vi "Lithographify.vi"(0 "interpolation distance":dbl, 1 "Path Settings.lvclass":refnum<class "Path Settings.lvclass">, 5 "Data In":cluster{string, cluster{"X":dbl, "Y":dbl}[]}, 7 "Direction":u16, 9 "Speed (um/s)":T1={"Schedule"=enum."Constant", "Settings"=variant(dbl 0.0)}, 11 "Voltage (V)":T1={"Schedule"=enum."Constant", "Settings"=variant(dbl 0.0)}, 13 "Enabled":bool) -> (4 "Lithography Data":T3)   [LabVIEW 2019]
doc: "This VI calculates the lithography data of one pattern and organizes it appropriately."
uses:
  typedefs/Voltage - cluster.ctl
  typedefs/Schedule - enum.ctl
  Classes/Settings/Path Settings/Path Settings.lvclass
  typedefs/Schedule Types/Schedule--Formula.ctl
  Classes/Settings/ObjectSettings/ObjectSettings.lvclass
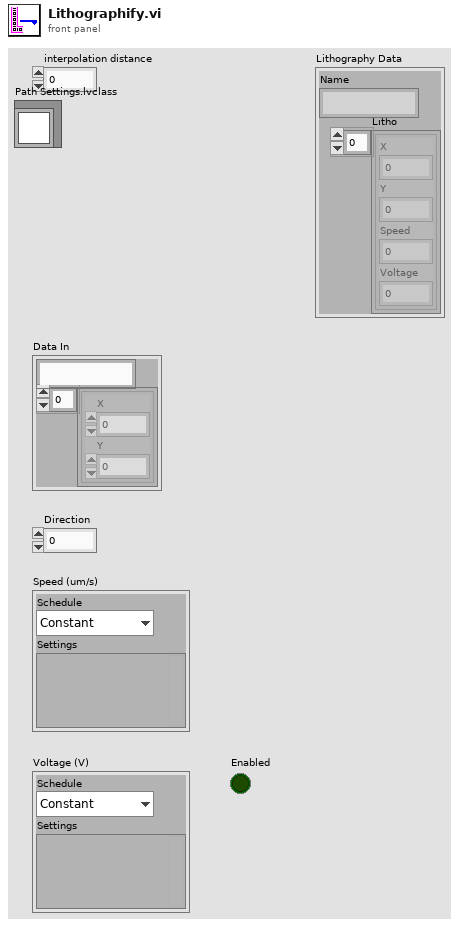
[diagram p1: front panel]
types:
  T1 = typedef "Voltage - cluster.ctl" = cluster{"Schedule":T2, "Settings":variant}
  T2 = typedef "Schedule - enum.ctl" = enum16{"Constant", "Ramp", "Fn. Generator", "Formula"}
  T3 = cluster{"Name":string, "Litho":cluster{"X":dbl, "Y":dbl, "Speed":dbl, "Voltage":dbl}[]}
  T4 = typedef "Schedule--Formula.ctl" = cluster{"formula":string, "formula length (nm)":dbl, "formula resolution (nm)":dbl}
  T5 = cluster{"X":dbl, "Y":dbl, "Speed":dbl, "Voltage":dbl}[]
  T6 = cluster{"X":dbl, "Y":dbl, "Speed":dbl, "Voltage":dbl}
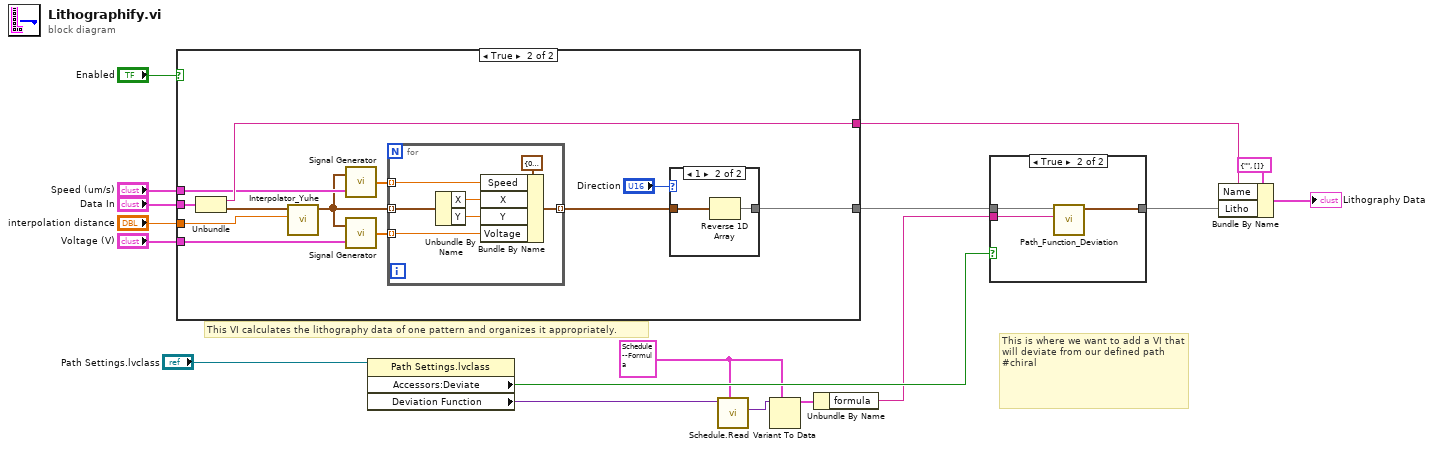
[diagram p0: block diagram]
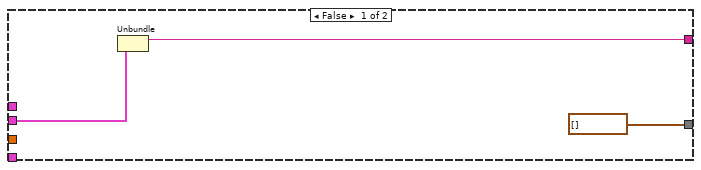
[diagram p3: hidden frame]
diagram:
  w5 = T4 {"formula"="1*(step(170-t)*cos(0.62831853071*t)+step(t-170)*cos(0.62831853071*(t-170))*(-1))", "formula length (nm)"=340.0, "formula resolution (nm)"=0.001} ("Formula")
  # "This is where we want to add a VI that will deviate from our defined path\n#chiral"
  # "This VI calculates the lithography data of one pattern and organizes it appropriately."
  n1 = case shown="True" "Enabled" {
    tunnel: [w20 w32] -> w8
    tunnel: "Data In" -> [w18 w31]
    tunnel: "Voltage (V)" -> [_ w28]
    tunnel: "Speed (um/s)" -> [_ w27]
    tunnel: [T5 [] w25] -> w10
    tunnel: "interpolation distance" -> [_ w21]
    frame False {
      n2 = Unbundle(w18) -> (w20:string)  [unwired: 1 out]
    }
    frame True {
      n3 = Unbundle(w31) -> (w32:string, w23:cluster{"X":dbl, "Y":dbl}[])
      n4 = call "Interpolator_Yuhe.vi"("interpolation distance"=w21, "Array in"=w23) -> ("Array out"=w22:cluster{"X":dbl, "Y":dbl}[])  [unwired: 9 in]
      n5 = call "Signal Generator.vi"("Signal Properties"=w27, "Points"=w22) -> ("Signal"=w29:dbl[])
      n6 = call "Signal Generator.vi"("Signal Properties"=w28, "Points"=w22) -> ("Signal"=w30:dbl[])
      n7 = for {
        tunnel: w29 -> [w36] mode=indexing
        tunnel: w30 -> [w38] mode=indexing
        tunnel: w22 -> [w40] mode=indexing
        tunnel: [w37] -> w26 mode=indexing
        n8 = Unbundle By Name(w40) -> ("X"=w41:dbl, "Y"=w39:dbl)
        n9 = Bundle By Name(cluster=T6 {"X"=0.0, "Y"=0.0, "Speed"=0.0, "Voltage"=0.0} ("Litho Point"), "Speed"=w36, "X"=w41, "Y"=w39, "Voltage"=w38) -> (w37:T6)
      }
      n10 = case shown="1" "Direction" {
        tunnel: w26 -> [w33 w35]
        tunnel: [w33 w34] -> w25
        frame 0, Default {
        }
        frame 1 {
          n11 = Reverse 1D Array(array=w35) -> (reversed array=w34:T5)
        }
      }
    }
  }
  n12 = property class="Path Settings.lvclass"(reference="Path Settings.lvclass") -> ("Accessors:Deviate"=w6:bool, "Deviation Function"=w2:variant)  [unwired: 1 in, 2 out]
  n13 = call "Schedule.Read.vi"("Data to Read"=w5, "LUT In"=w2) -> ("Data Out"=w4:variant)  [unwired: 7 in, 2 out]
  n14 = Variant To Data(type=w5, Variant=w4) -> (data=w3:T4)  [unwired: 1 in, 1 out]
  n15 = Unbundle By Name(w3) -> ("formula"=w1:string)
  n16 = case shown="True" w6 {
    tunnel: w10 -> [w43 w46]
    tunnel: [w43 w45] -> w9
    tunnel: w1 -> [_ w44]
    frame False {
    }
    frame True {
      n17 = call "Path_Function_Deviation.vi"("Function In"=w44, "Path Points In"=w46) -> ("Path Points Out"=w45:T5)  [unwired: 9 in]
    }
  }
  n18 = Bundle By Name(cluster=T3 {"Name"="", "Litho"=[]} ("Lithography Data"), "Name"=w8, "Litho"=w9) -> (→"Lithography Data":T3)
